vi "Message Window Dialog Box with Sound.vi"(1 "sound? (F)":bool, 2 "modality (0)":i32(ring) items=["Application", "System", "Task"], 3 "icon (0:None)":i32(ring), 4 "buttons (0:OK)":i32(ring), 5 "message (\"\")":string, 6 "window title (\"\")":string) -> (0 "button pressed":i32(ring) items=["OK", "CANCEL", "ABORT", "RETRY", "IGNORE", "YES", "NO"])   [LabVIEW 2023, in "Winevent.lvlib"]
doc: "This VI calls the Windows functions MessageBox and MessageBeep to display a message dialog box and, optionally, play a sound effect. These functions are in the Windows DLL called USER.EXE, which is located in the windows\\system directory. If your computer is not equipped with a sound driver, a short \"beep\" will be played through the PC's speaker.\n\nVarious combinations of dialog boxes are possible. The buttons input selects which buttons are displayed in the dialog box, the icon input determines the icon, if any, and the modality box determines whether the dialog box is system, application, or task modal.\n\nThe following dialog box button schemes are available through the \"buttons\" input:\n0: OK\n1: OK / Cancel\n2: Abort / Retry / Ignore\n3: Yes / No / Cancel\n4: Yes / No\n5: Retry / Cancel\n\nThe following icons are available through the \"icon\" input:\n0: None\n1: STOP icon\n2: Question icon\n3: Exclamation icon\n4: Information icon\n\nThe following three modalities are available:\n0: Application\n1: System\n2: Task\n\nIf sounds are enabled, the icon option determines the sound effect played, as defined in the Sounds section of Windows' Control Panel.\n\nThe DLL functions called are:\n\nint MessageBox ( hWndParent, lpText, lpCaption, wType )\nvoid MessageBeep ( wType )\n\nFunction definitions are from:\nMicrosoft Windows Programmer's Reference\nCopyright 1990 Microsoft Corporation."
uses:
  Winevent.lvlib
  user32.dll
panel:
  in  "buttons":i32[](array[numeric])=[0, 1, 2, 3, 4, 5, 16, 32, 48, 64] format="%.0x"
  in  "icons":i32[](array[numeric])=[0, 16, 32, 48, 64, 5, 16, 32, 48, 64] format="%.0x"
  in  "modal constants":i32[](array[numeric])=[0, 4096, 8192] format="%.0x"
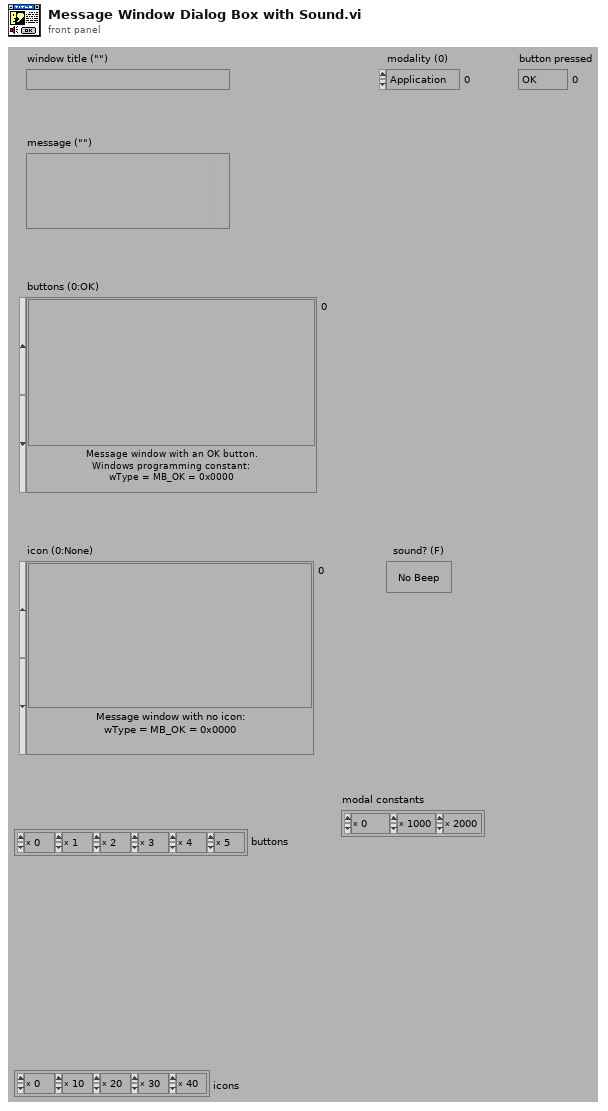
[diagram p1: front panel]
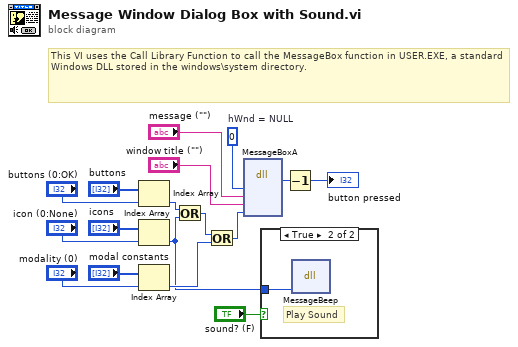
[diagram p0: block diagram]
diagram:
  w16 = u32 0  # hWnd = NULL
  # "This VI uses the Call Library Function to call the MessageBox function in USER.EXE, a standard Windows DLL stored in the windows\\system directory."
  n1 = Index Array(array="buttons", index="buttons (0:OK)") -> (element=w4:i32)
  n2 = Index Array(array="icons", index="icon (0:None)") -> (element=w1:i32)
  n3 = Index Array(array="modal constants", index="modality (0)") -> (element=w3:i32)
  n4 = Or(x=w4, y=w1) -> (x .or. y?=w2:i32)
  n5 = Or(x=w2, y=w3) -> (x .or. y?=w8:i32)
  n6 = dll-call lib="USER32.DLL" fn="MessageBoxA" label="MessageBox"("hWndParent"=w16, "lpText"="message (\"\")", "lpCaption"="window title (\"\")", "wType"=w8) -> (w13:i32)  [unwired: 7 in, 2 out]
  n7 = case shown="True" "sound? (F)" {
    tunnel: w1 -> [_ w18]
    frame False {
      # "Do not play sound effects."
    }
    frame True {
      # "Play Sound"
      n8 = dll-call lib="USER32.DLL" fn="MessageBeep"("wType"=w18) -> ()  [unwired: 4 in, 3 out]
    }
  }
  n9 = Decrement(x=w13) -> (x-1=→"button pressed":i32)
